vi "GitDoCmd.vi"(5 "standard input":string, 7 "error in (no error)":errorcluster, 8 "Working Path":path=path "", 9 "Git command":string, 10 "Git exec":string="git") -> (0 "error out":errorcluster, 1 "Working Path out":path, 2 "Returned stdout":string, 3 "Git exec out":string)   [LabVIEW 2013]
uses:
  <vilib>/dlg_ctls.llb/Space Constant.vi
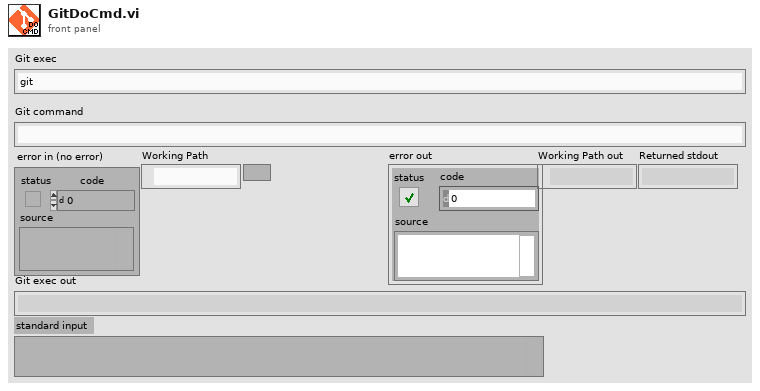
[diagram p1: front panel]
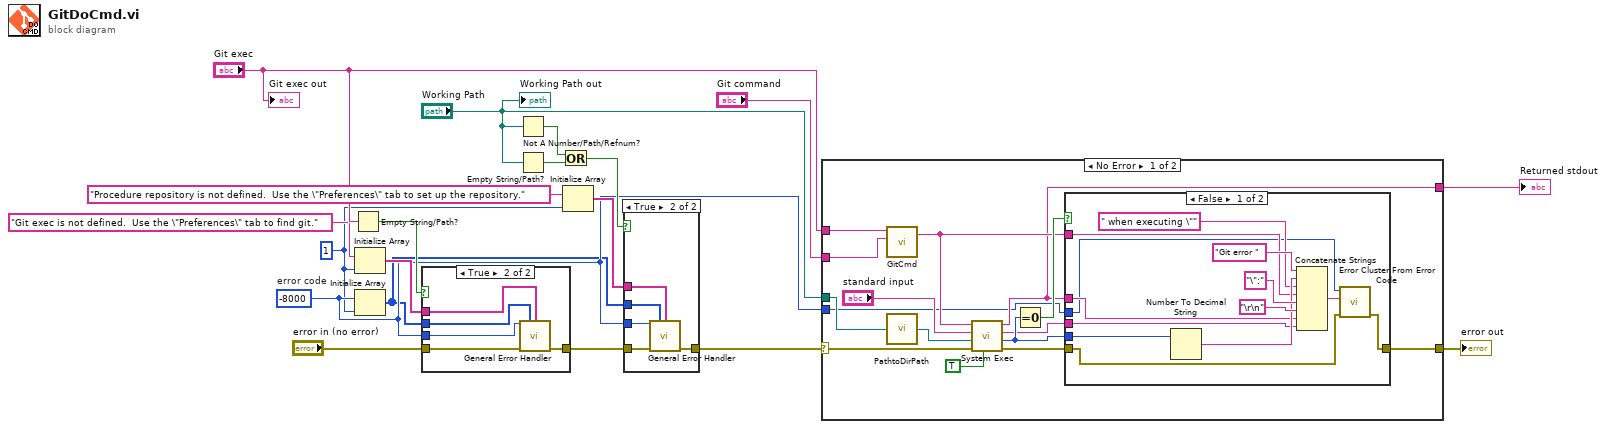
[diagram p0: block diagram]
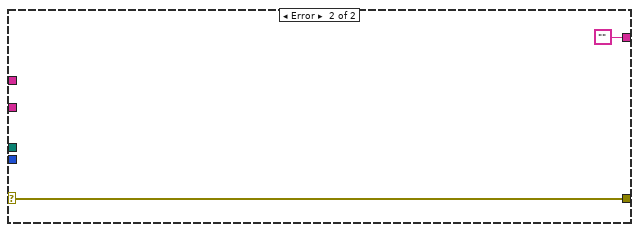
[diagram p5: hidden frame]
diagram:
  w1 = 1 ("dimension size")
  w3 = -8000  # error code
  n1 = Empty String/Path?(string/path="Git exec") -> (empty?=w12:bool)
  n2 = Initialize Array("Git exec is not defined.  Use the \"Preferences\" tab to find git." ("error message (\"\")"), w1) -> (w6:string[])
  n3 = Initialize Array(w3, w1) -> (w2:i32[])
  n4 = case shown="True" w12 {
    tunnel: "error in (no error)" -> [w20 w25]
    tunnel: [w20 w24] -> w9
    tunnel: w3 -> [_ w23]
    tunnel: w6 -> [_ w22]
    tunnel: w2 -> [_ w21]
    frame False {
    }
    frame True {
      n5 = call <vilib>:"General Error Handler.vi"("[error code] (0)"=w23, "[user-defined codes]"=w21, "[user-defined descriptions]"=w22, "error in (no error)"=w25) -> ("error out"=w24:errorcluster)  [unwired: 7 in, 4 out]
    }
  }
  n6 = Not A Number/Path/Refnum?(number/path/refnum="Working Path") -> (NaN/Path/Refnum?=w14:bool)
  n7 = Empty String/Path?(string/path="Working Path") -> (empty?=w15:bool)
  n8 = Or(x=w14, y=w15) -> (x .or. y?=w11:bool)
  n9 = Initialize Array("Procedure repository is not defined.  Use the \"Preferences\" tab to set up the repository." ("error message (\"\")"), w1) -> (w4:string[])
  n10 = case shown="True" w11 {
    tunnel: w9 -> [w26 w30]
    tunnel: [w26 w31] -> w8
    tunnel: w3 -> [_ w29]
    tunnel: w4 -> [_ w28]
    tunnel: w2 -> [_ w27]
    frame False {
    }
    frame True {
      n11 = call <vilib>:"General Error Handler.vi"("[error code] (0)"=w29, "[user-defined codes]"=w27, "[user-defined descriptions]"=w28, "error in (no error)"=w30) -> ("error out"=w31:errorcluster)  [unwired: 7 in, 4 out]
    }
  }
  n12 = case shown="No Error" w8 {
    selector: w8 -> [w43 w61]
    tunnel: "Git exec" -> [w46 _]
    tunnel: "Git command" -> [w45 _]
    tunnel: "Working Path" -> [w44 _]
    tunnel: [w37 w61] -> w18
    tunnel: [w33 ""] -> w17
    tunnel: w3 -> [w32 _]
    frame No Error {
      n13 = call "GitCmd.vi"("Git command"=w45, "Git exec"=w46) -> ("Cmd output"=w35:string)  [unwired: 3 in]
      n14 = call "PathtoDirPath.vi"("Path"=w44) -> ("Path out"=w41:path)
      n15 = call <vilib>:"System Exec.vi"("run minimized? (F)"=TRUE, "error in (no error)"=w43, "working directory"=w41, "standard input"="standard input", "command line"=w35) -> ("error out"=w40:errorcluster, "return code"=w38:i32, "standard error"=w36:string, "standard output"=w33:string)  [unwired: 3 in]
      n16 = Equal To 0?(x=w38) -> (x = 0?=w39:bool)
      n17 = case shown="False" w39 {
        tunnel: w40 -> [w59 w60]
        tunnel: w38 -> [w57 _]
        tunnel: w36 -> [w52 _]
        tunnel: [w58 w60] -> w37
        tunnel: w35 -> [w49 _]
        tunnel: w33 -> [w48 _]
        tunnel: w32 -> [w47 _]
        frame False {
          n18 = Number To Decimal String(number=w57) -> (decimal integer string=w53:string)  [unwired: 1 in]
          n19 = Concatenate Strings("Git error " ("string"), w53, " when executing \"" ("string"), w49, "\":" ("string"), "\r\n", w48, w52) -> (w51:string)
          n20 = call <vilib>:"Error Cluster From Error Code.vi"("error in (no error)"=w59, "error message (\"\")"=w51, "error code (0)"=w47) -> ("error out"=w58:errorcluster)  [unwired: 6 in]
        }
        frame True {
        }
      }
    }
    frame Error {
    }
  }
  "error out" <- w18
  "Returned stdout" <- w17
  "Working Path out" <- "Working Path"
  "Git exec out" <- "Git exec"
